vi "Find All Minima nD.vi"(0 "gradient method":u16(ring) items=["Fletcher-Reeves", "Polak-Ribiere"], 1 "algorithm":u16(ring) items=["Conjugate Gradient", "Downhill Simplex"], 2 "accuracy":dbl=1e-08 format="%.2e", 5 "line minimum":u16(ring) items=["without derivatives", "with derivatives"], 7 "number of trials":i32=5, 9 "Start":dbl[](array[numeric]) format="%.2f", 11 "End":dbl[](array[numeric]) format="%.2f", 12 "X":string[](array[string]), 13 "F(X)":string) -> (4 "X Values":dbl[][](array[numeric]) format="%.2f", 6 "F Values":dbl[](array[numeric]) format="%.2f", 8 "ticks":u32, 10 "error":i32)   [LabVIEW 2014, in "NI_Gmath.lvlib"]
doc: "Determines the minima of an n-dimension function in a given n-dimension interval."
uses:
  NI_Gmath.lvlib
panel:
  # "only for Conjugate Gradient"
  # "Example:\n\n accuracy: 1E-8\n algorithm: Conjugate Gradient \n gradient method: Fletcher-Reeves \n line minimum: without derivatives \n number of trials: 5 \n Start: 0.0 and 0.0 \n End: 1.0 and 1.0\n X: x and y\n F(X): x^2+y^2+sin(x-y)"
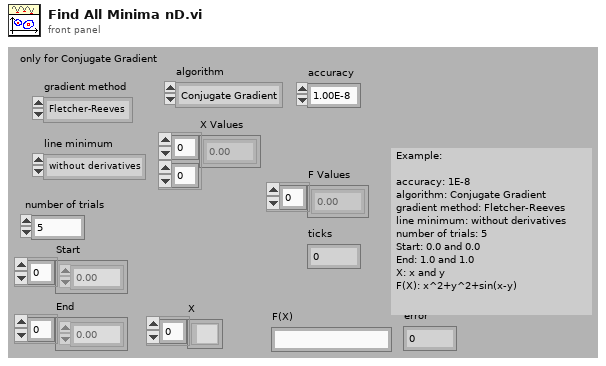
[diagram p1: front panel]
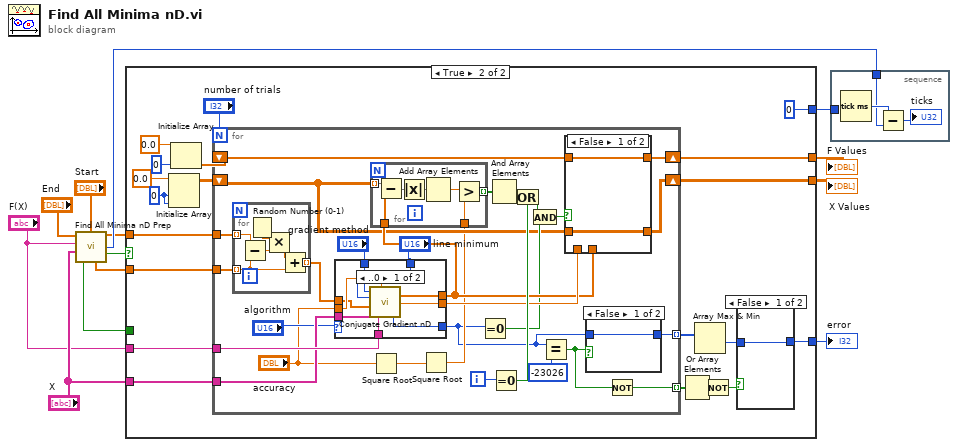
[diagram p0: block diagram]
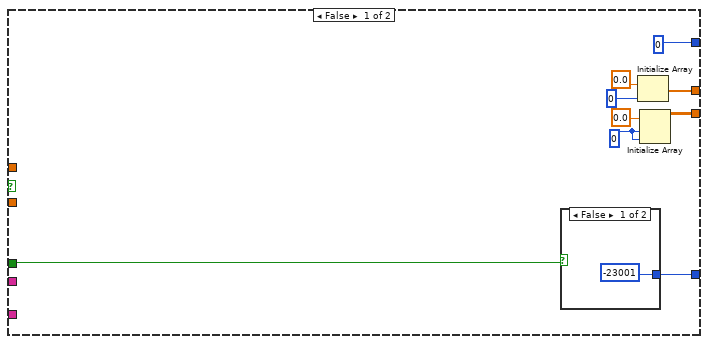
[diagram p2: hidden frame]
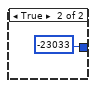
[diagram p3: hidden frame]
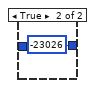
[diagram p4: hidden frame]
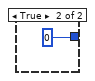
[diagram p5: hidden frame]
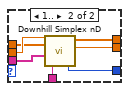
[diagram p6: hidden frame]
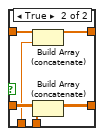
[diagram p7: hidden frame]
diagram:
  n1 = call "Find All Minima nD Prep.vi"("Start"="Start", "X"="X", "F(X)"="F(X)", "End"="End") -> ("error (general)"=w5:bool, "Start"=w7:dbl[], "time [msec]"=w12:u32, "End"=w6:dbl[], "specific error"=w4:bool)
  n2 = case shown="True" w5 {
    tunnel: [0 0] -> w13
    tunnel: "X" -> [_ w42]
    tunnel: "F(X)" -> [_ w41]
    tunnel: [w17 w34] -> w10
    tunnel: [w16 w33] -> w9
    tunnel: [w15 w31] -> w8
    tunnel: w7 -> [_ w30]
    tunnel: w6 -> [_ w29]
    tunnel: w4 -> [w14 _]
    frame False {
      w18 = 0
      n3 = case shown="False" w14 {
        tunnel: [-23001 -23033] -> w15
        frame False {
        }
        frame True {
        }
      }
      n4 = Initialize Array(0.0, 0) -> (w17:dbl[])
      n5 = Initialize Array(0.0, w18, w18) -> (w16:dbl[][])
    }
    frame True {
      w36 = 0
      n6 = Initialize Array(0.0, w36, w36) -> (w35:dbl[][])
      n7 = Initialize Array(0.0, 0) -> (w38:dbl[])
      n8 = for {
        N: "number of trials" -> [_]
        tunnel: w29 -> [w75]
        tunnel: w30 -> [w74]
        tunnel: w42 -> [w68]
        tunnel: w41 -> [w69]
        shift-right: [w64] -> w34
        shift-left: w38 -> [w72]
        shift-right: [w65] -> w33
        shift-left: w35 -> [w53]
        tunnel: [w55] -> w32 mode=indexing
        tunnel: [w48] -> w27 mode=indexing
        i -> [w51]
        n9 = for {
          tunnel: w75 -> [w114] mode=indexing
          tunnel: w74 -> [w111] mode=indexing
          tunnel: [w109] -> w67 mode=indexing
          n10 = Subtract(x=w114, y=w111) -> (x-y=w113:dbl)
          n11 = Random Number (0-1)() -> (number: 0 to 1=w112:dbl)
          n12 = Multiply(x=w112, y=w113) -> (x*y=w110:dbl)
          n13 = Add(x=w110, y=w111) -> (x+y=w109:dbl)
        }
        n14 = case shown="..0" "algorithm" {
          tunnel: [w84 w93] -> w66
          tunnel: w67 -> [w80 w88]
          tunnel: "accuracy" -> [w81 w89]
          tunnel: w68 -> [w79 w92]
          tunnel: w69 -> [w86 w91]
          tunnel: [w85 w90] -> w61
          tunnel: "line minimum" -> [w82 _]
          tunnel: "gradient method" -> [w83 _]
          tunnel: [w78 w87] -> w49
          frame ..0 {
            n15 = call "Conjugate Gradient nD.vi"("f(X)"=w86, "accuracy"=w81, "X"=w79, "Start"=w80, "line minimization"=w82, "gradient method"=w83) -> ("error"=w78:i32, "f(Minimum)"=w84:dbl, "Minimum"=w85:dbl[])  [unwired: 1 out]
          }
          frame 1.. {
            n16 = call "Downhill Simplex nD.vi"("f(X)"=w91, "X"=w92, "Start"=w88, "accuracy"=w89) -> ("error"=w87:i32, "f(Minimum)"=w93:dbl, "Minimum"=w90:dbl[])  [unwired: 1 out]
          }
        }
        n17 = Square Root(x="accuracy") -> (sqrt(x)=w50:dbl)
        n18 = Square Root(x=w50) -> (sqrt(x)=w52:dbl)
        n19 = for {
          tunnel: w53 -> [w108] mode=indexing
          tunnel: [w104] -> w73 mode=indexing
          tunnel: w52 -> [w105]
          tunnel: w61 -> [w103]
          n20 = Subtract(x=w108, y=w103) -> (x-y=w107:dbl[])
          n21 = Absolute Value(x=w107) -> (abs(x)=w106:dbl[])
          n22 = Add Array Elements(numeric array=w106) -> (sum=w102:dbl)
          n23 = Greater?(x=w102, y=w105) -> (0:w104:bool)
        }
        n24 = Equal To 0?(x=w49) -> (x = 0?=w58:bool)
        n25 = And Array Elements(Boolean array=w73) -> (logical AND=w70:bool)
        n26 = Equal To 0?(x=w51) -> (x = 0?=w71:bool)
        n27 = Or(x=w70, y=w71) -> (x .or. y?=w59:bool)
        n28 = And(x=w59, y=w58) -> (x .and. y?=w57:bool)
        n29 = Equal?(x=w49, y=-23026) -> (x = y?=w54:bool)
        n30 = case shown="False" w57 {
          tunnel: w72 -> [w95 w99]
          tunnel: [w95 w98] -> w64
          tunnel: w53 -> [w94 w101]
          tunnel: [w94 w100] -> w65
          tunnel: w61 -> [_ w97]
          tunnel: w66 -> [_ w96]
          frame False {
          }
          frame True {
            n31 = Build Array (concatenate)(w99, w96) -> (w98:dbl[])
            n32 = Build Array (concatenate)(w101, w97) -> (w100:dbl[][])
          }
        }
        n33 = case shown="False" w54 {
          tunnel: w49 -> [w76 _]
          tunnel: [w76 0] -> w55
          frame False {
          }
          frame True {
          }
        }
        n34 = Not(x=w54) -> (.not. x?=w48:bool)
      }
      n35 = Or Array Elements(Boolean array=w27) -> (logical OR=w26:bool)
      n36 = Array Max & Min(array=w32) -> (min value=w28:i32)  [unwired: 3 out]
      n37 = Not(x=w26) -> (.not. x?=w25:bool)
      n38 = case shown="False" w25 {
        tunnel: [w45 -23026] -> w31
        tunnel: w28 -> [w45 _]
        frame False {
        }
        frame True {
        }
      }
    }
  }
  "error" <- w8
  "F Values" <- w10
  "X Values" <- w9
  n39 = stacked-sequence {
    tunnel: w12 -> [w116]
    tunnel: w13 -> [_]
    frame #0 {
      n40 = Tick Count (ms)() -> (millisecond timer value=w117:u32)
      n41 = Subtract(x=w117, y=w116) -> (x-y=→"ticks":u32)
    }
  }
